vi "PTScanner.panel.vi"(0 "object ref":refnum<vi>, 5 "error in (no error)":errorcluster) -> ()   [LabVIEW 2014, in "PTScanner.lvlib"]
doc: "This is the front panel VI for the PTScanner class.\n\ndescriptionHelpStart\nThe PTScanner class has been designed to be used interactively by a normal user. The main aim of this class is to provide a possibility of multi-dimensional scan for any integer or floating-point single value among the CS system.\n\nAt first, user has to add values to be scanned and to organize them in the corresponding order. Each value is represented by several parameters:\n- object\n- \"set\" method (can have many parameters)\n- method parameters (with one of them to be scanned)\n- central point\n- \"minus\" and \"plus\" values (start point is a difference between \"central\" and \"minus\" values, stop point is a sum of \"central\" and \"plus\" respectively)\n- step size\n- call mode which means how will be realized the movement from one step to the next one. The check of nominal (from current step) and actual values conformity can be done in a simple mode (here you should know the corresponding service) or in a synchronous mode (assuming that the method has a feedback of excatly the same parameters as input parameters)\n- as an option one can input service address for the synchronization directly. Do it only if you know exactly what is it!!!\n\nAfter the list of values is formed you have to form the scan sequence. You can check the scan sequence by \"View -> Scan Table\" from the window menu (have to wait some time before the representation table will be formed). Now you can run your scan in two modes: single (sequence will be runned only once) and loop (sequence will be runned continuously).\n\nDelay is a delay time (in ms) between two steps.\ndescriptionHelpStop\n\nLicense Agreement for the PTScanner class:\n\nCopyright (C)\nMikhail Goncharov\nMax-Planck-Institut fuer Kernphysik\nSaupfercheckweg 1\n69117 Heidelberg\nGermany\n\nContact: mikhail.goncharov@mpi-hd.mpg.de\n\nThis program is free software; you can redistribute it and/or modify it under the terms of the GNU General Public License as published by the Free Software Foundation; either version 2 of the license, or (at your option) any later version.\n\nThis program is distributed in the hope that it will be useful, but WITHOUT ANY WARRANTY; without even the implied warranty of MERCHANTABILITY or FITNESS FOR A PARTICULAR PURPOSE. See the GNU General License for more details (http://www.gnu.org).\n\nLast update: 2-DEC-2010\n\n\nmenuHelpStart\nFile\n==\n- \"Load\" loads a list of values to be scanned. After that you have to form a scan.\n\n- \"Save/Save As\" saves the actual list of values.\n\n- \"Hide\" just hides this GUI (but it remains alive in the background).\n\n- \"Close\" closes this window and removes this process from the system.\n\nOperate\n=====\n- \"Start\" starts scan sequence. Awailable only after the sequence is formed.\n\n- \"Pause\" pauses current run. Awailable only during the running of the sequence.\n\n- \"Stop\" stops scan sequence.\n\n- \"Reset\" resets the scanner (sets the first step as a current and nulls all counters).\n\n- \"Reset Values\" sets all variables to their central values.\n\nView\n=====\n- \"Scan Table\" forms and shows the representation of the current formed scan sequence. If there are a lot of steps and values it could take some time so be patient =)\nmenuHelpStop"
uses:
  PTScanner.lvlib
  CSlibraries/UtilityLib/UtilityLib.helpType.ctl
  CSCore/CSSystem/CoreLib/CoreLib.string 2 byte array.vi
  CSCore/CSSystem/CSSystemLib/CSSystemLib.lvlib
  CSlibraries/UtilityLib/UtilityLib.lvlib
  _common/PTUtils/PTUtils.lvlib
  CSCore/CSSystem/CoreLib/CoreLib.lvlib
  CSCore/BaseProcess/BaseProcess.lvlib
  CSCore/BaseSM/BaseSM.lvlib
  CSCore/CSObj/CSObj.lvlib
panel:
  in  "Form step list":bool
  out "NewValue":i32
  out "state":string caption="State:"
  in  "Scan Delay":u32 caption="Delay:"
  out "Paused":bool
  in  "Set previous step":bool
  in  "Set next step":bool
  out "Current step":i32 caption="Step"
  in  "Mode":u16(ring) caption="Mode:" items=["Single", "Loop"]
  out "All done":bool caption="Done"
  out "Running":bool
  out "OldValue":i32
  in  "settings path":path caption="Settings file"
  out "Busy":bool
  out "ErrorString":string
  in  "tab":enum32{"Objects", "Scan Tree"}(tab)
  in  "object list":i32(listbox)
  out "Status Log":string
  out "Steps":string(tree)
  out "loop counter":i32
  out "error out":errorcluster
  # "ms"
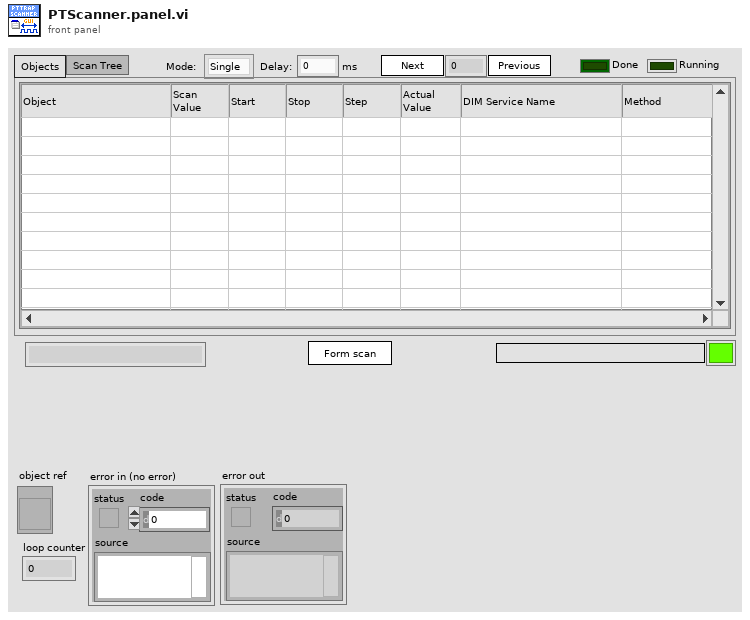
[diagram p1: front panel]
types:
  T1 = enum8{"Enabled", "Disabled", "Disabled and Grayed Out"}
  T2 = enum16{"open", "replace", "create", "open or create", "replace or create", "replace or create with confirmation"}
  T3 = typedef "UtilityLib.lvlib/UtilityLib.helpType.ctl" = enum16{"unknown", "menu", "description", "about", "special0", "special1", "special2"}
  T4 = typedef "BaseProcess.lvlib/BaseProcess.i attribute.ctl" = cluster{"EventStatus":string, "EventError":i32, "PresetEvtWatchD":i32, "PresetPdcWatchD":i32, "EventTimeout":i32, "PeriodicInterval":i32, "Interface":string[], "Address":string[], "Special":string[], "PeriodicError":i32, "PeriodicStatus":string, "SuperProc":string, "Descriptors":T5[], "CaseRef":refnum<vi>, "PdcRef":refnum<vi>, "Thread Ref":refnum<vi>, "eventErrorID":i32, "eventStatusID":i32, "periodicErrorID":i32, "periodicStatusID":i32, "pdcCtrID":i32}
  T5 = typedef "BaseProcess.lvlib/BaseProcess.descriptor definition.ctl" = cluster{"selector":string, "descriptor":T6}
  T6 = typedef "BaseProcess.lvlib/BaseProcess.descriptor string definition.ctl" = string
  T7 = typedef "PTScanner.lvlib/PTScanner.i attribute.ctl" = cluster{"Object cmds":T8[], "Steps":cluster{"Finished":bool, "cmd setup":T9[]}[], "curStep":i32, "DIM IDs":cluster{"AllFinished":i32, "Finished":i32, "curStep":i32, "nofSteps":i32, "NomValues":i32[], "1D-Min":i32, "1D-Max":i32, "Dimensions":i32, "MaxDimensions":i32, "ScanedDeviceNames":i32[]}, "All Finished":bool, "DIMs in use":string[], "Running":bool, "Scan Delay":u32, "loop":bool, "Paused":bool, "Formed":bool}
  T8 = typedef "PTScanner.lvlib/PTScanner.obj parameters.ctl" = cluster{"object":string, "DIM address":string, "method":string, "data descriptor":string, "method parameters":cluster{"Name":string, "Descr":string, "Value":string, "Value?":bool}[], "Call Mode":enum16{"Simple DIM", "Synchronous"}, "actValue":dbl, "Centroid":dbl, "Minus Delta":dbl, "Plus Delta":dbl, "increment":dbl, "DIM Status":cluster{"no link":bool, "quality":i32, "Time Stamp":timestamp}, "range":dbl, "DIMChannelIndex":i32}
  T9 = typedef "PTScanner.lvlib/PTScanner.step obj parameters.ctl" = cluster{"obj index":i32, "nomValue":dbl, "fulfilled":bool}
  T10 = cluster{"Name":string, "Descr":string, "Value":string, "Value?":bool}[]
  T11 = typedef "CoreDefs.rawDataType.ctl" = i8[]
  T12 = typedef "eventvkey.ctl" = enum16{"ASCII", "Enter", "Return", "Shift", "Ctrl", "Alt", "Cmd", "Opt", "Caps", "NumLock", "Clear", "Break", "Up", "Down", "Left", "Right", "Insert", "Delete", "Home", "End", "PageUp", "PageDown", "Escape", "Help", "Pause", "ScrollLock", "F1", "F2", "F3", "F4", "F5", "F6", "F7", "F8", "F9", "F10", "F11", "F12", "F13", "F14", "F15", "F16", "F17", "F18", "F19", "F20", "F21", "F22", "F23", "F24", "Play", "VolumeUp", "VolumeDown", "Mute", "Two Byte Char"}
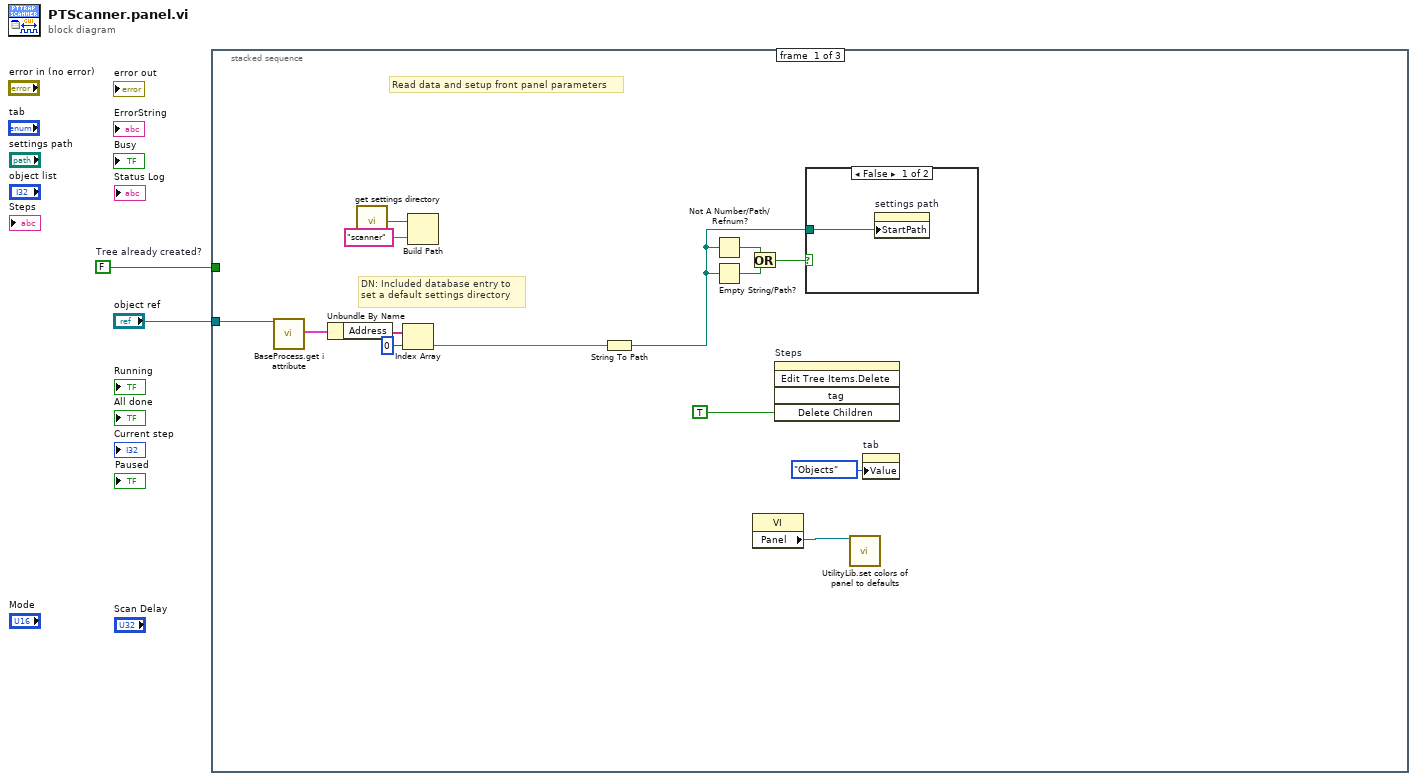
[diagram p0: block diagram]
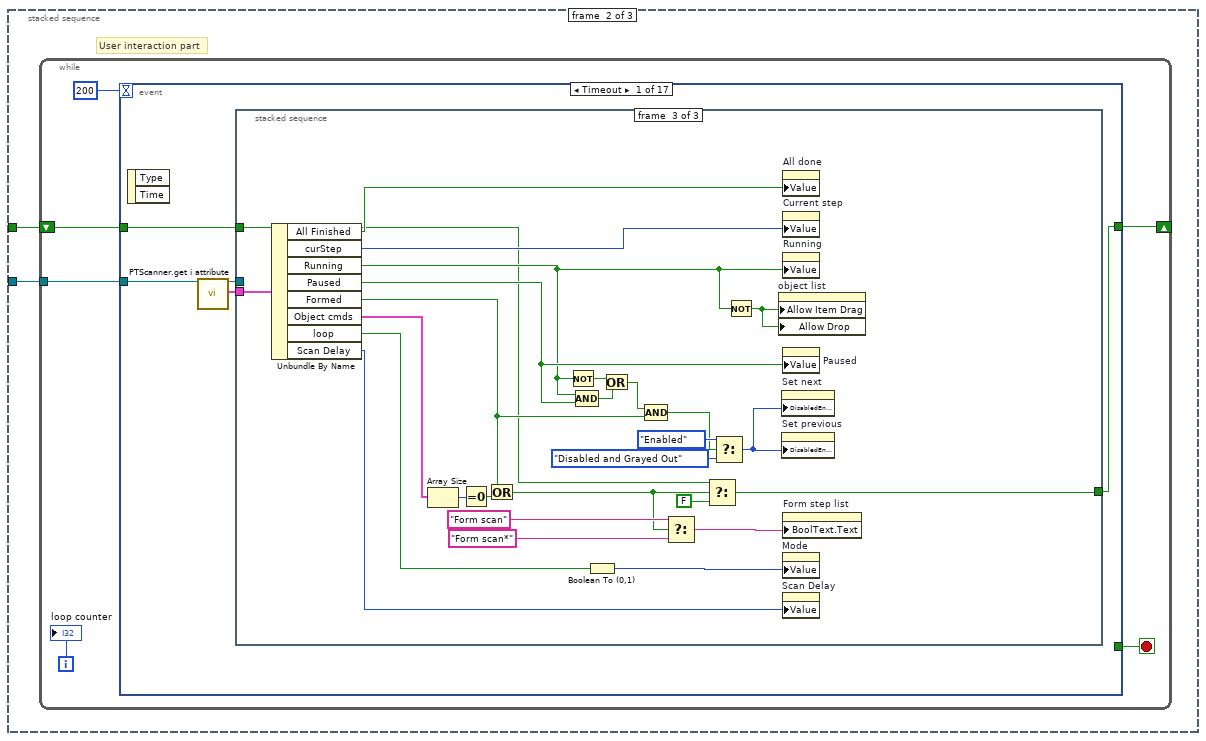
[diagram p3: hidden frame]
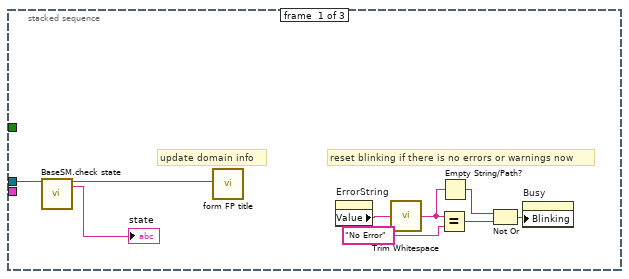
[diagram p4: hidden frame]
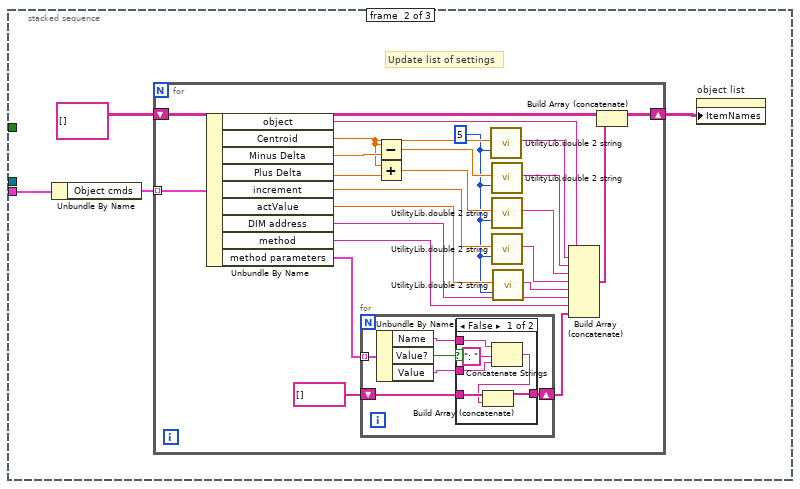
[diagram p5: hidden frame]
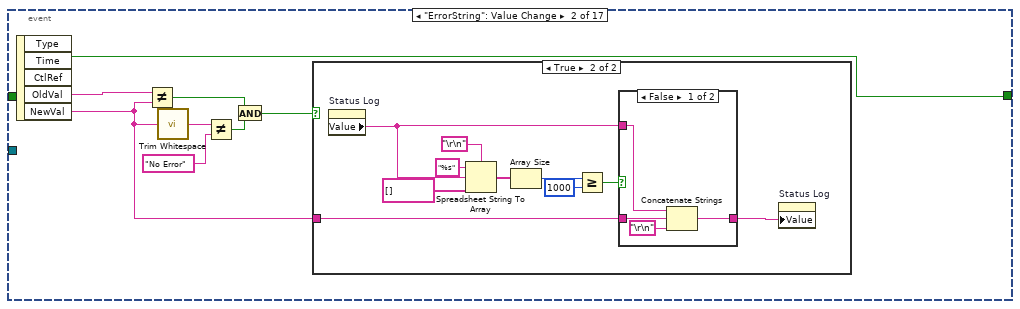
[diagram p7: hidden frame]
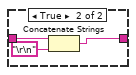
[diagram p9: hidden frame]
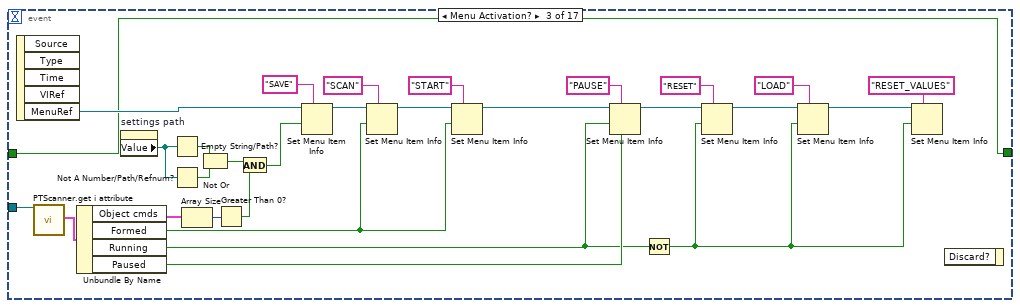
[diagram p10: hidden frame]
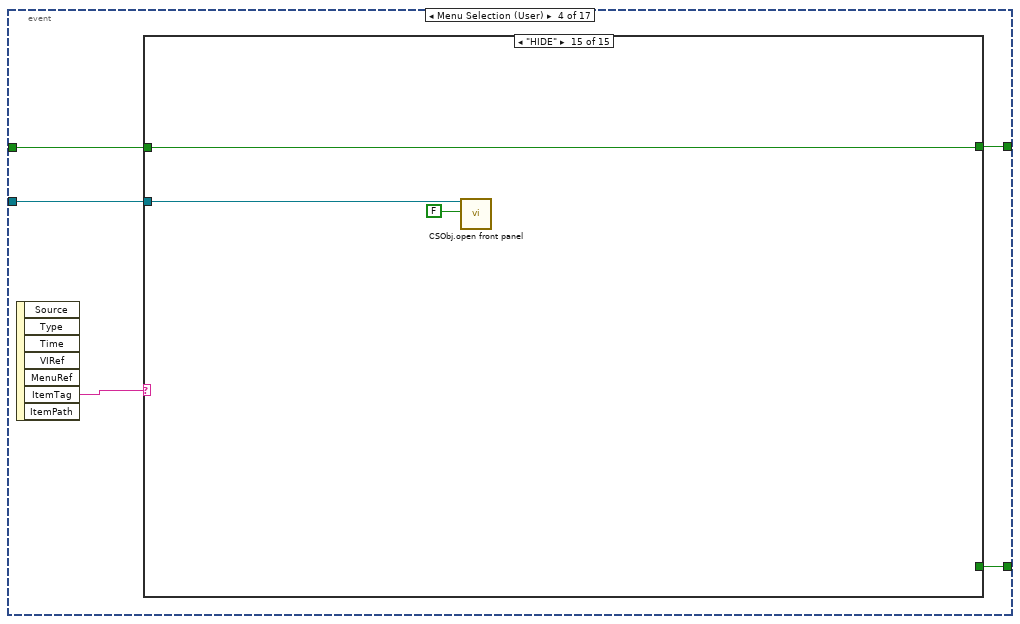
[diagram p11: hidden frame]
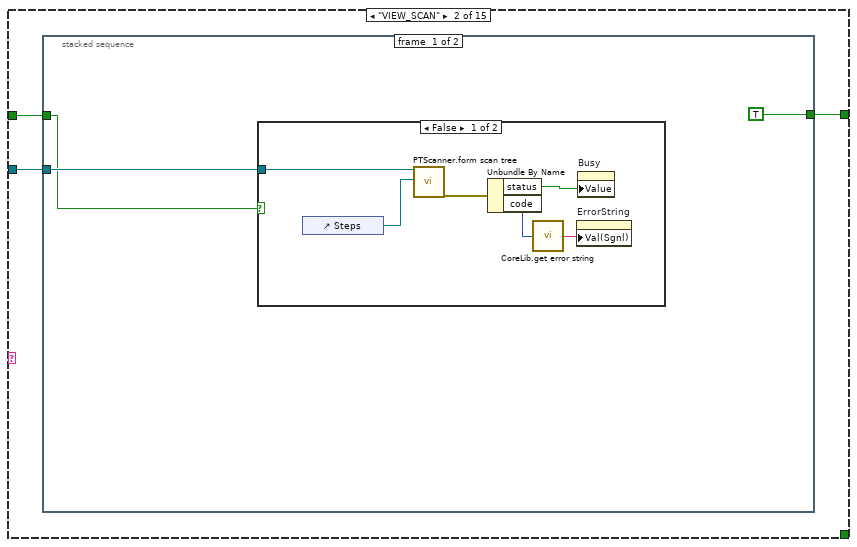
[diagram p13: hidden frame]
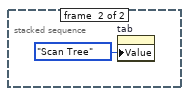
[diagram p15: hidden frame]
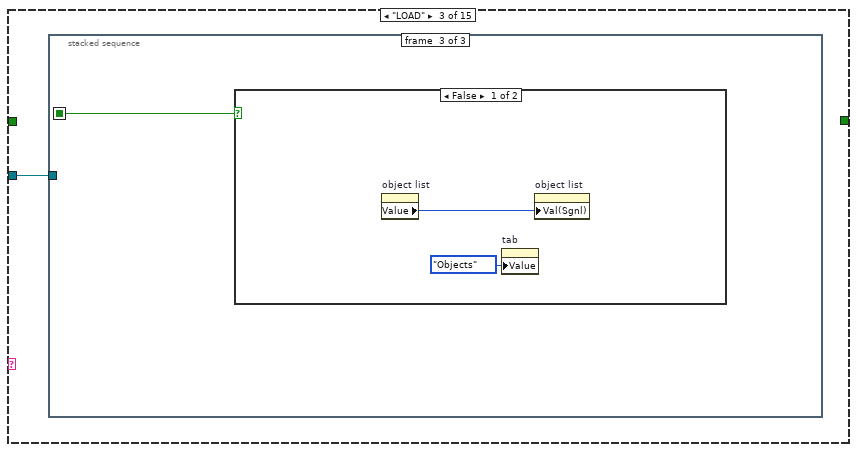
[diagram p16: hidden frame]
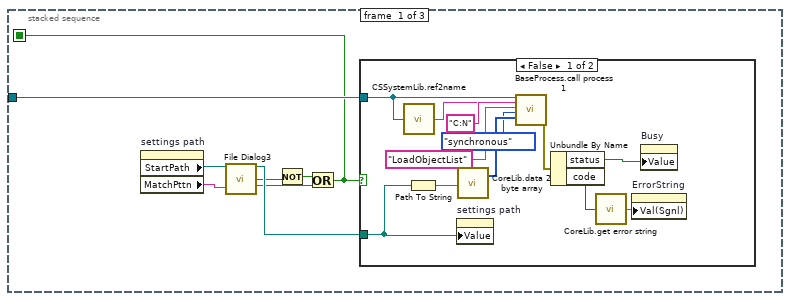
[diagram p17: hidden frame]
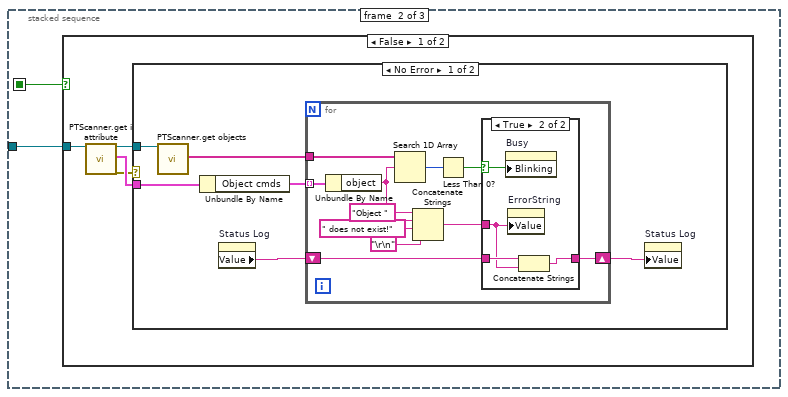
[diagram p19: hidden frame]
diagram:
  w1 = FALSE  # Tree already created?
  n1 = stacked-sequence {
    tunnel: "object ref" -> [w8 w19 w550]
    tunnel: w1 -> [_ w18 _]
    frame #0 {
      # "DN: Included database entry to\nset a default settings directory"
      # "Read data and setup front panel parameters"
      n2 = call "BaseProcess.get i attribute.vi"("i ref in"=w8) -> ("i attribute"=w7:T4)  [unwired: 16 in, 2 out]
      n3 = Unbundle By Name(w7) -> ("Address"=w6:string[])
      n4 = call "get settings directory.vi"() -> ("settings directory"=w12:path)
      n5 = Index Array(array=w6, index=0) -> (element=w4:string)
      n6 = Build Path(base path=w12, name or relative path="scanner") -> ()  [unwired: 1 out]
      n7 = String To Path(string=w4) -> (path=w3:path)
      n8 = Not A Number/Path/Refnum?(number/path/refnum=w3) -> (NaN/Path/Refnum?=w15:bool)
      n9 = Empty String/Path?(string/path=w3) -> (empty?=w14:bool)
      n10 = Or(x=w15, y=w14) -> (x .or. y?=w13:bool)
      n11 = property class="VI"() -> ("Panel"=w10:refnum<vi>)  [unwired: 2 in, 2 out]
      n12 = invoke on="Steps" class="Tree (strict)" method="Edit Tree Items.Delete"("Delete Children"=TRUE) -> ()  [unwired: 4 in, 5 out]
      n13 = case shown="False" w13 {
        tunnel: w3 -> [w17 _]
        frame False {
          n14 = property on="settings path" class="Path"("StartPath"=w17) -> ()  [unwired: 2 in, 2 out]
        }
        frame True {
        }
      }
      n15 = call "UtilityLib.set colors of panel to defaults.vi"("Front Panel"=w10) -> ()  [unwired: 18 in, 1 out]
      n16 = property on="tab" class="TabCtl (strict)"("Value"=enum32{"Objects", "Scan Tree"}."Objects" ("tab")) -> ()  [unwired: 2 in, 2 out]
    }
    frame #1 {
      # "User interaction part"
      n17 = while {
        tunnel: w19 -> [w25]
        shift-right: [w20] -> _
        shift-left: w18 -> [w21]
        i -> [w23]
        stop <- w22 stop-if-true
        n18 = event shown="[0] Timeout" {
          selector: _ -> [_ _ _ _ _ _ _ _ _ _ _ _ _ _ _ _ _]
          dyn-events: _ -> [_ _ _ _ _ _ _ _ _ _ _ _ _ _ _ _ _]
          timeout: 200 -> [_ _ _ _ _ _ _ _ _ _ _ _ _ _ _ _ _]
          tunnel: w25 -> [w30 _ w155 w164 w335 w353 _ w366 w398 w403 w468 w490 w517 w520 w528 w540 w547]
          tunnel: [_ _ _ w163 _ _ _ _ _ _ _ _ _ _ _ _ _] -> w22
          tunnel: w21 -> [w27 w107 w132 w162 w334 w342 w361 w364 w386 w402 w466 w489 _ w518 w526 w534 w546]
          tunnel: [w26 w107 w132 w161 TRUE w342 w361 w364 w386 w402 w466 w489 TRUE w518 w526 w534 w546] -> w20
          event Timeout {
            n19 = event-data() -> ()  [unwired: 1 in, 2 out]
            n20 = call "PTScanner.get i attribute.vi"("i ref in"=w30) -> ("i ref out"=w28:refnum<vi>, "i attribute"=w29:T7)  [unwired: 16 in, 1 out]
            n21 = stacked-sequence {
              tunnel: w29 -> [_ w41 w103]
              tunnel: w28 -> [w33 _ _]
              tunnel: w27 -> [_ _ w82]
              tunnel: [_ _ w80] -> w26
              frame #0 {
                # "update domain info"
                # "reset blinking if there is no errors or warnings now"
                n22 = call "BaseSM.check state.vi"("i ref in"=w33) -> ("i ref out"=w32:refnum<vi>, "actualState"=→"state":string)  [unwired: 13 in, 4 out]
                n23 = call "form FP title.vi"("object ref"=w32) -> ()  [unwired: 19 in]
                n24 = property on="ErrorString" class="Str"() -> ("Value"=w39:string)  [unwired: 2 in, 2 out]
                n25 = call <vilib>:"Trim Whitespace.vi"("string"=w39) -> ("trimmed string"=w37:string)  [unwired: 1 in]
                n26 = Equal?(x=w37, y="No Error") -> (x = y?=w35:bool)
                n27 = Empty String/Path?(string/path=w37) -> (empty?=w36:bool)
                n28 = Not Or(1:w35, 2:w36) -> (0:w34:bool)
                n29 = property on="Busy" class="Bool (strict)"("Blinking"=w34) -> ()  [unwired: 2 in, 2 out]
              }
              frame #1 {
                # "Update list of settings"
                n30 = Unbundle By Name(w41) -> ("Object cmds"=w42:T8[])
                n31 = for {
                  tunnel: w42 -> [w66] mode=indexing
                  shift-right: [w51] -> w40
                  shift-left: string[][] [] -> [w52]
                  w53 = u8 5
                  n32 = Unbundle By Name(w66) -> ("object"=w48:string, "Centroid"=w63:dbl, "Minus Delta"=w65:dbl, "Plus Delta"=w62:dbl, "increment"=w60:dbl, "actValue"=w59:dbl, "DIM address"=w54:string, "method"=w47:string, "method parameters"=w46:T10)
                  n33 = for {
                    tunnel: w46 -> [w72] mode=indexing
                    shift-right: [w70] -> w44
                    shift-left: string[] [] -> [w71]
                    n34 = Unbundle By Name(w72) -> ("Name"=w67:string, "Value?"=w68:bool, "Value"=w69:string)
                    n35 = case shown="False" w68 {
                      tunnel: w71 -> [w78 w79]
                      tunnel: [w77 w79] -> w70
                      tunnel: w67 -> [w76 _]
                      tunnel: w69 -> [w74 _]
                      frame False {
                        n36 = Concatenate Strings(w76, ": ", w74) -> (w73:string)
                        n37 = Build Array (concatenate)(w78, w73) -> (w77:string[])
                      }
                      frame True {
                      }
                    }
                  }
                  n38 = Subtract(x=w63, y=w65) -> (x-y=w64:dbl)
                  n39 = Add(x=w63, y=w62) -> (x+y=w61:dbl)
                  n40 = call "UtilityLib.double 2 string.vi"("Numeric"=w63, "length"=w53) -> ("String"=w49:string)  [unwired: 16 in, 1 out]
                  n41 = call "UtilityLib.double 2 string.vi"("Numeric"=w64, "length"=w53) -> ("String"=w58:string)  [unwired: 16 in, 1 out]
                  n42 = call "UtilityLib.double 2 string.vi"("Numeric"=w61, "length"=w53) -> ("String"=w57:string)  [unwired: 16 in, 1 out]
                  n43 = call "UtilityLib.double 2 string.vi"("Numeric"=w60, "length"=w53) -> ("String"=w56:string)  [unwired: 16 in, 1 out]
                  n44 = call "UtilityLib.double 2 string.vi"("Numeric"=w59, "length"=w53) -> ("String"=w55:string)  [unwired: 16 in, 1 out]
                  n45 = Build Array (concatenate)(w48, w49, w58, w57, w56, w55, w54, w47, w44) -> (w50:string[])
                  n46 = Build Array (concatenate)(w52, w50) -> (w51:string[][])
                }
                n47 = property on="object list" class="MCListbox (strict)"("ItemNames"=w40) -> ()  [unwired: 2 in, 2 out]
              }
              frame #2 {
                n48 = Unbundle By Name(w103) -> ("All Finished"=w92:bool, "curStep"=w93:i32, "Running"=w85:bool, "Paused"=w88:bool, "Formed"=w90:bool, "Object cmds"=w99:T8[], "loop"=w96:bool, "Scan Delay"=w94:u32)
                n49 = Array Size(array=w99) -> (size(s)=w98:i32)
                n50 = Equal To 0?(x=w98) -> (x = 0?=w97:bool)
                n51 = Or(x=w90, y=w97) -> (x .or. y?=w83:bool)
                n52 = Not(x=w85) -> (.not. x?=w89:bool)
                n53 = Compound Arithmetic op=AND(w85, w88) -> (w87:bool)
                n54 = Boolean To (0,1)(Boolean=w96) -> (0, 1=w95:i16)
                n55 = Or(x=w89, y=w87) -> (x .or. y?=w86:bool)
                n56 = Compound Arithmetic op=AND(w86, w90) -> (w91:bool)
                n57 = Select(t="Form scan", s=w83, f="Form scan*") -> (s? t:f=w102:string)
                n58 = Select(t=w82, s=w83, f=FALSE) -> (s? t:f=w80:bool)
                n59 = Select(t=T1."Enabled" ("Disabled"), s=w91, f=T1."Disabled and Grayed Out" ("Disabled")) -> (s? t:f=w106:T1)
                n60 = Not(x=w85) -> (.not. x?=w84:bool)
                n61 = property on="object list" class="MCListbox (strict)"("Allow Item Drag"=w84, "Allow Drop"=w84) -> ()  [unwired: 2 in, 2 out]
                n62 = property on="Set next" class="Bool"("DisabledEnum"=w106) -> ()  [unwired: 2 in, 2 out]
                n63 = property on="Set previous" class="Bool"("DisabledEnum"=w106) -> ()  [unwired: 2 in, 2 out]
                n64 = property on="All done" class="Bool (strict)"("Value"=w92) -> ()  [unwired: 2 in, 2 out]
                n65 = property on="Current step" class="DigNum (strict)"("Value"=w93) -> ()  [unwired: 2 in, 2 out]
                n66 = property on="Running" class="Bool (strict)"("Value"=w85) -> ()  [unwired: 2 in, 2 out]
                n67 = property on="Paused" class="Bool (strict)"("Value"=w88) -> ()  [unwired: 2 in, 2 out]
                n68 = property on="Form step list" class="Bool"("BoolText.Text"=w102) -> ()  [unwired: 2 in, 2 out]
                n69 = property on="Mode" class="Ring (strict)"("Value"=w95) -> ()  [unwired: 2 in, 2 out]
                n70 = property on="Scan Delay" class="DigNum (strict)"("Value"=w94) -> ()  [unwired: 2 in, 2 out]
              }
            }
          }
          event "ErrorString": Value Change {
            n71 = event-data() -> ("OldVal"=w114:string, "NewVal"=w111:string)  [unwired: 1 in, 3 out]
            n72 = Not Equal?(x=w114, y=w111) -> (x != y?=w109:bool)
            n73 = call <vilib>:"Trim Whitespace.vi"("string"=w111) -> ("trimmed string"=w113:string)  [unwired: 1 in]
            n74 = Not Equal?(x=w113, y="No Error") -> (x != y?=w110:bool)
            n75 = And(x=w109, y=w110) -> (x .and. y?=w108:bool)
            n76 = case shown="True" w108 {
              tunnel: w111 -> [_ w116]
              frame False {
              }
              frame True {
                n77 = property on="Status Log" class="Str"() -> ("Value"=w117:string)  [unwired: 2 in, 2 out]
                n78 = Spreadsheet String To Array(delimiter (Tab)="\r\n", format string="%s", spreadsheet string=w117, array type (2D Dbl)=string[] []) -> (array=w121:string[])
                n79 = Array Size(array=w121) -> (size(s)=w120:i32)
                n80 = Greater Or Equal?(x=w120, y=1000) -> (x >= y?=w118:bool)
                n81 = case shown="False" w118 {
                  tunnel: w117 -> [w128 _]
                  tunnel: w116 -> [w127 w130]
                  tunnel: [w125 w129] -> w115
                  frame False {
                    n82 = Concatenate Strings(w128, w127, "\r\n") -> (w125:string)
                  }
                  frame True {
                    n83 = Concatenate Strings(w130, "\r\n") -> (w129:string)
                  }
                }
                n84 = property on="Status Log" class="Str"("Value"=w115) -> ()  [unwired: 2 in, 2 out]
              }
            }
          }
          event Menu Activation? {
            n85 = event-data() -> ("MenuRef"=w160:refnum<k9>)  [unwired: 1 in, 4 out]
            n86 = call "PTScanner.get i attribute.vi"("i ref in"=w155) -> ("i attribute"=w154:T7)  [unwired: 16 in, 2 out]
            n87 = Unbundle By Name(w154) -> ("Object cmds"=w153:T8[], "Formed"=w134:bool, "Running"=w142:bool, "Paused"=w145:bool)
            n88 = property on="settings path" class="Path"() -> ("Value"=w156:path)  [unwired: 2 in, 2 out]
            n89 = Empty String/Path?(string/path=w156) -> (empty?=w158:bool)
            n90 = Not A Number/Path/Refnum?(number/path/refnum=w156) -> (NaN/Path/Refnum?=w157:bool)
            n91 = Array Size(array=w153) -> (size(s)=w152:i32)
            n92 = Not Or(1:w157, 2:w158) -> (0:w150:bool)
            n93 = Greater Than 0?(x=w152) -> (x > 0?=w151:bool)
            n94 = And(x=w150, y=w151) -> (x .and. y?=w149:bool)
            n95 = Set Menu Item Info(7:"SAVE", 9:w149, 11:w160) -> (3:w148:refnum<k9>)  [unwired: 4 in, 1 out]
            n96 = Set Menu Item Info(7:"SCAN", 9:w134, 11:w148) -> (3:w135:refnum<k9>)  [unwired: 4 in, 1 out]
            n97 = Set Menu Item Info(7:"START", 9:w134, 11:w135) -> (3:w133:refnum<k9>)  [unwired: 4 in, 1 out]
            n98 = Set Menu Item Info(6:w145, 7:"PAUSE", 9:w142, 11:w133) -> (3:w143:refnum<k9>)  [unwired: 3 in, 1 out]
            n99 = Not(x=w142) -> (.not. x?=w137:bool)
            n100 = Set Menu Item Info(7:"RESET", 9:w137, 11:w143) -> (3:w140:refnum<k9>)  [unwired: 4 in, 1 out]
            n101 = Set Menu Item Info(7:"LOAD", 9:w137, 11:w140) -> (3:w138:refnum<k9>)  [unwired: 4 in, 1 out]
            n102 = Set Menu Item Info(7:"RESET_VALUES", 9:w137, 11:w138) -> ()  [unwired: 4 in, 2 out]
            n103 = event-data() -> ()  [unwired: 2 in, 1 out]
          }
          event Menu Selection (User) {
            n104 = event-data() -> ("ItemTag"=w165:string)  [unwired: 1 in, 6 out]
            n105 = case shown="\"HIDE\"" w165 {
              tunnel: w164 -> [_ w169 w180 w237 w257 _ w282 w290 w302 w310 w318 _ _ _ w331]
              tunnel: [_ _ _ _ _ TRUE _ _ _ _ _ _ _ _ _] -> w163
              tunnel: w162 -> [w166 w168 _ w236 w255 w279 w281 w289 w297 w308 w316 w324 w326 w328 w330]
              tunnel: [w166 w167 _ w236 w255 w279 w281 w289 w297 w308 w316 w324 w326 w328 w330] -> w161
              frame "", Default {
              }
              frame "VIEW_SCAN" {
                n106 = stacked-sequence {
                  tunnel: w169 -> [w172 _]
                  tunnel: w168 -> [w171 _]
                  tunnel: [TRUE _] -> w167
                  frame #0 {
                    n107 = case shown="False" w171 {
                      tunnel: w172 -> [w177 _]
                      frame False {
                        n108 = control-ref of="Steps"() -> (w178:refnum<vi>)
                        n109 = call "PTScanner.form scan tree.vi"("VI Refnum"=w177, "Scan Tree Ref"=w178) -> ("error out"=w173:errorcluster)  [unwired: 16 in, 1 out]
                        n110 = Unbundle By Name(w173) -> ("status"=w176:bool, "code"=w174:i32)
                        n111 = call "CoreLib.get error string.vi"("Error Code"=w174) -> ("Error String"=w175:string)
                        n112 = property on="ErrorString" class="Str"("Val(Sgnl)"=w175) -> ()  [unwired: 2 in, 2 out]
                        n113 = property on="Busy" class="Bool (strict)"("Value"=w176) -> ()  [unwired: 2 in, 2 out]
                      }
                      frame True {
                      }
                    }
                  }
                  frame #1 {
                    n114 = property on="tab" class="TabCtl (strict)"("Value"=enum32{"Objects", "Scan Tree"}."Scan Tree" ("tab")) -> ()  [unwired: 2 in, 2 out]
                  }
                }
              }
              frame "LOAD" {
                n115 = stacked-sequence {
                  seq-local: [w182 _ _] -> [_ w201 w233]
                  tunnel: w180 -> [w186 w202 _]
                  frame #0 {
                    n116 = property on="settings path" class="Path"() -> ("StartPath"=w188:path, "MatchPttn"=w187:string)  [unwired: 2 in, 2 out]
                    n117 = call "File Dialog3"("start path"=w188, "pattern (all files)"=w187) -> ("selected path"=w185:path, "exists"=w181:bool, "cancelled"=w183:bool)  [unwired: 10 in, 1 out]
                    n118 = Not(x=w181) -> (.not. x?=w184:bool)
                    n119 = Or(x=w184, y=w183) -> (x .or. y?=w182:bool)
                    n120 = case shown="False" w182 {
                      tunnel: w186 -> [w192 _]
                      tunnel: w185 -> [w190 _]
                      frame False {
                        n121 = call "CSSystemLib.ref2name.vi"("obj refnum"=w192) -> ("name"=w193:string)
                        n122 = Path To String(path=w190) -> (string=w191:string)
                        n123 = property on="settings path" class="Path"("Value"=w190) -> ()  [unwired: 2 in, 2 out]
                        n124 = call-poly "CoreLib.data 2 byte array.vi"("string"=w191) -> ("byteArray out"=w194:T11)  [unwired: 18 in]
                        n125 = call "BaseProcess.call process 1.vi"("i ref in"=w192, "Object"=w193, "Selector"="LoadObjectList", "CallType"=enum16{"simple", "synchronous", "asynchronous"}."synchronous", "Data"=w194, "Data Descriptor"="C:N") -> ("error out"=w197:errorcluster)  [unwired: 11 in, 2 out]
                        n126 = Unbundle By Name(w197) -> ("status"=w200:bool, "code"=w198:i32)
                        n127 = call "CoreLib.get error string.vi"("Error Code"=w198) -> ("Error String"=w199:string)
                        n128 = property on="ErrorString" class="Str"("Val(Sgnl)"=w199) -> ()  [unwired: 2 in, 2 out]
                        n129 = property on="Busy" class="Bool (strict)"("Value"=w200) -> ()  [unwired: 2 in, 2 out]
                      }
                      frame True {
                      }
                    }
                  }
                  frame #1 {
                    n130 = case shown="False" w201 {
                      tunnel: w202 -> [w204 _]
                      frame False {
                        n131 = call "PTScanner.get i attribute.vi"("i ref in"=w204) -> ("i ref out"=w203:refnum<vi>, "i attribute"=w206:T7, "error out"=w205:errorcluster)  [unwired: 16 in]
                        n132 = case shown="No Error" w205 {
                          selector: w205 -> [_ w229]
                          tunnel: w206 -> [w210 _]
                          tunnel: w203 -> [w208 _]
                          frame No Error {
                            n133 = call "PTScanner.get objects.vi"("i ref in"=w208) -> ("objects"=w207:string[])  [unwired: 18 in]
                            n134 = Unbundle By Name(w210) -> ("Object cmds"=w209:T8[])
                            n135 = property on="Status Log" class="Str"() -> ("Value"=w212:string)  [unwired: 2 in, 2 out]
                            n136 = for {
                              tunnel: w209 -> [w222] mode=indexing
                              tunnel: w207 -> [w223]
                              shift-right: [w213] -> w211
                              shift-left: w212 -> [w215]
                              n137 = Unbundle By Name(w222) -> ("object"=w219:string)
                              n138 = Search 1D Array(1D array=w223, element=w219) -> (index of element=w221:i32)  [unwired: 1 in]
                              n139 = Concatenate Strings("Object ", w219, " does not exist!", "\r\n") -> (w214:string)
                              n140 = Less Than 0?(x=w221) -> (x < 0?=w220:bool)
                              n141 = case shown="True" w220 {
                                selector: w220 -> [_ w225]
                                tunnel: w215 -> [w224 w228]
                                tunnel: w214 -> [_ w227]
                                tunnel: [w224 w226] -> w213
                                frame False {
                                }
                                frame True {
                                n142 = property on="Busy" class="Bool (strict)"("Blinking"=w225) -> ()  [unwired: 2 in, 2 out]
                                n143 = property on="ErrorString" class="Str"("Value"=w227) -> ()  [unwired: 2 in, 2 out]
                                n144 = Concatenate Strings(w228, w227) -> (w226:string)
                                }
                              }
                            }
                            n145 = property on="Status Log" class="Str"("Value"=w211) -> ()  [unwired: 2 in, 2 out]
                          }
                          frame Error {
                            n146 = Unbundle By Name(w229) -> ("status"=w232:bool, "code"=w230:i32)
                            n147 = call "CoreLib.get error string.vi"("Error Code"=w230) -> ("Error String"=w231:string)
                            n148 = property on="ErrorString" class="Str"("Val(Sgnl)"=w231) -> ()  [unwired: 2 in, 2 out]
                            n149 = property on="Busy" class="Bool (strict)"("Value"=w232) -> ()  [unwired: 2 in, 2 out]
                          }
                        }
                      }
                      frame True {
                      }
                    }
                  }
                  frame #2 {
                    n150 = case shown="False" w233 {
                      frame False {
                        n151 = property on="object list" class="MCListbox (strict)"() -> ("Value"=w235:i32)  [unwired: 2 in, 2 out]
                        n152 = property on="tab" class="TabCtl (strict)"("Value"=enum32{"Objects", "Scan Tree"}."Objects" ("tab")) -> ()  [unwired: 2 in, 2 out]
                        n153 = property on="object list" class="MCListbox (strict)"("Val(Sgnl)"=w235) -> ()  [unwired: 2 in, 2 out]
                      }
                      frame True {
                      }
                    }
                  }
                }
              }
              frame "SAVE" {
                n154 = property on="settings path" class="Path"() -> ("Value"=w240:path)  [unwired: 2 in, 2 out]
                n155 = Open/Create/Replace File(file path (use dialog)=w240, operation (0:open)=T2."replace or create", access (0:read/write)=enum16{"read/write", "read-only", "write-only"}."read-only") -> (refnum out=w241:refnum<file>, cancelled=w243:bool)  [unwired: 3 in, 1 out]
                n156 = Close File(refnum=w241) -> (path=w242:path)  [unwired: 1 in, 1 out]
                n157 = case shown="False" w243 {
                  tunnel: w242 -> [w244 _]
                  tunnel: w237 -> [w246 _]
                  frame False {
                    n158 = call "CSSystemLib.ref2name.vi"("obj refnum"=w246) -> ("name"=w245:string)
                    n159 = Path To String(path=w244) -> (string=w247:string)
                    n160 = property on="settings path" class="Path"("Value"=w244) -> ()  [unwired: 2 in, 2 out]
                    n161 = call-poly "CoreLib.data 2 byte array.vi"("string"=w247) -> ("byteArray out"=w248:T11)  [unwired: 18 in]
                    n162 = call "BaseProcess.call process 2.vi"("i ref in"=w246, "Object"=w245, "Selector"="SaveObjectList", "Data Descriptor"="C:N", "Data"=w248) -> ("error out"=w251:errorcluster)  [unwired: 13 in, 1 out]
                    n163 = Unbundle By Name(w251) -> ("status"=w254:bool, "code"=w252:i32)
                    n164 = call "CoreLib.get error string.vi"("Error Code"=w252) -> ("Error String"=w253:string)
                    n165 = property on="Busy" class="Bool (strict)"("Value"=w254) -> ()  [unwired: 2 in, 2 out]
                    n166 = property on="ErrorString" class="Str"("Val(Sgnl)"=w253) -> ()  [unwired: 2 in, 2 out]
                  }
                  frame True {
                  }
                }
              }
              frame "SAVE_AS" {
                n167 = property on="settings path" class="Path"() -> ("StartPath"=w260:path, "MatchPttn"=w259:string)  [unwired: 2 in, 2 out]
                n168 = call "File Dialog4"("start path"=w260, "pattern (all files)"=w259) -> ("selected path"=w258:path, "cancelled"=w256:bool)  [unwired: 10 in, 2 out]
                n169 = case shown="False" w256 {
                  tunnel: w258 -> [w266 _]
                  tunnel: w257 -> [w267 _]
                  frame False {
                    n170 = Open/Create/Replace File(file path (use dialog)=w266, operation (0:open)=T2."replace or create with confirmation", access (0:read/write)=enum16{"read/write", "read-only", "write-only"}."read-only") -> (refnum out=w265:refnum<file>, cancelled=w263:bool)  [unwired: 3 in, 1 out]
                    n171 = Close File(refnum=w265) -> (path=w264:path)  [unwired: 1 in, 1 out]
                    n172 = case shown="False" w263 {
                      tunnel: w264 -> [w268 _]
                      tunnel: w267 -> [w270 _]
                      frame False {
                        n173 = call "CSSystemLib.ref2name.vi"("obj refnum"=w270) -> ("name"=w269:string)
                        n174 = Path To String(path=w268) -> (string=w271:string)
                        n175 = property on="settings path" class="Path"("Value"=w268) -> ()  [unwired: 2 in, 2 out]
                        n176 = call-poly "CoreLib.data 2 byte array.vi"("string"=w271) -> ("byteArray out"=w272:T11)  [unwired: 18 in]
                        n177 = call "BaseProcess.call process 2.vi"("i ref in"=w270, "Object"=w269, "Selector"="SaveObjectList", "Data Descriptor"="C:N", "Data"=w272) -> ("error out"=w275:errorcluster)  [unwired: 13 in, 1 out]
                        n178 = Unbundle By Name(w275) -> ("status"=w278:bool, "code"=w276:i32)
                        n179 = call "CoreLib.get error string.vi"("Error Code"=w276) -> ("Error String"=w277:string)
                        n180 = property on="ErrorString" class="Str"("Val(Sgnl)"=w277) -> ()  [unwired: 2 in, 2 out]
                        n181 = property on="Busy" class="Bool (strict)"("Value"=w278) -> ()  [unwired: 2 in, 2 out]
                      }
                      frame True {
                      }
                    }
                  }
                  frame True {
                  }
                }
              }
              frame "QUIT" {
              }
              frame "START" {
                n182 = call "CSSystemLib.ref2name.vi"("obj refnum"=w282) -> ("name"=w283:string)
                n183 = call "BaseProcess.call process 2.vi"("i ref in"=w282, "Object"=w283, "Selector"="Start") -> ("error out"=w284:errorcluster)  [unwired: 15 in, 1 out]
                n184 = Unbundle By Name(w284) -> ("status"=w287:bool, "code"=w285:i32)
                n185 = call "CoreLib.get error string.vi"("Error Code"=w285) -> ("Error String"=w286:string)
                n186 = property on="ErrorString" class="Str"("Val(Sgnl)"=w286) -> ()  [unwired: 2 in, 2 out]
                n187 = property on="Busy" class="Bool (strict)"("Value"=w287) -> ()  [unwired: 2 in, 2 out]
              }
              frame "STOP" {
                n188 = call "CSSystemLib.ref2name.vi"("obj refnum"=w290) -> ("name"=w291:string)
                n189 = call "BaseProcess.call process 2.vi"("i ref in"=w290, "Object"=w291, "Selector"="Stop") -> ("error out"=w292:errorcluster)  [unwired: 15 in, 1 out]
                n190 = Unbundle By Name(w292) -> ("status"=w295:bool, "code"=w293:i32)
                n191 = call "CoreLib.get error string.vi"("Error Code"=w293) -> ("Error String"=w294:string)
                n192 = property on="ErrorString" class="Str"("Val(Sgnl)"=w294) -> ()  [unwired: 2 in, 2 out]
                n193 = property on="Busy" class="Bool (strict)"("Value"=w295) -> ()  [unwired: 2 in, 2 out]
              }
              frame "PAUSE" {
                n194 = call "CSSystemLib.ref2name.vi"("obj refnum"=w302) -> ("name"=w303:string)
                n195 = property on="Paused" class="Bool (strict)"() -> ("Value"=w298:bool)  [unwired: 2 in, 2 out]
                n196 = Select(t="Start", s=w298, f="Pause") -> (s? t:f=w299:string)
                n197 = call "BaseProcess.call process 2.vi"("i ref in"=w302, "Object"=w303, "Selector"=w299) -> ("error out"=w304:errorcluster)  [unwired: 15 in, 1 out]
                n198 = Unbundle By Name(w304) -> ("status"=w307:bool, "code"=w305:i32)
                n199 = call "CoreLib.get error string.vi"("Error Code"=w305) -> ("Error String"=w306:string)
                n200 = property on="ErrorString" class="Str"("Val(Sgnl)"=w306) -> ()  [unwired: 2 in, 2 out]
                n201 = property on="Busy" class="Bool (strict)"("Value"=w307) -> ()  [unwired: 2 in, 2 out]
              }
              frame "RESET" {
                n202 = call "CSSystemLib.ref2name.vi"("obj refnum"=w310) -> ("name"=w311:string)
                n203 = call "BaseProcess.call process 2.vi"("i ref in"=w310, "Object"=w311, "Selector"="Reset") -> ("error out"=w312:errorcluster)  [unwired: 15 in, 1 out]
                n204 = Unbundle By Name(w312) -> ("status"=w315:bool, "code"=w313:i32)
                n205 = call "CoreLib.get error string.vi"("Error Code"=w313) -> ("Error String"=w314:string)
                n206 = property on="ErrorString" class="Str"("Val(Sgnl)"=w314) -> ()  [unwired: 2 in, 2 out]
                n207 = property on="Busy" class="Bool (strict)"("Value"=w315) -> ()  [unwired: 2 in, 2 out]
              }
              frame "RESET_VALUES" {
                n208 = call "CSSystemLib.ref2name.vi"("obj refnum"=w318) -> ("name"=w319:string)
                n209 = call "BaseProcess.call process 2.vi"("i ref in"=w318, "Object"=w319, "Selector"="SetCentralValues") -> ("error out"=w320:errorcluster)  [unwired: 15 in, 1 out]
                n210 = Unbundle By Name(w320) -> ("status"=w323:bool, "code"=w321:i32)
                n211 = call "CoreLib.get error string.vi"("Error Code"=w321) -> ("Error String"=w322:string)
                n212 = property on="ErrorString" class="Str"("Val(Sgnl)"=w322) -> ()  [unwired: 2 in, 2 out]
                n213 = property on="Busy" class="Bool (strict)"("Value"=w323) -> ()  [unwired: 2 in, 2 out]
              }
              frame "helpOnMenus" {
                n214 = call "UtilityLib.show help.vi"("helpType"=UtilityLib.helpType."menu") -> ()
              }
              frame "helpDescription" {
                n215 = call "UtilityLib.show help.vi"("helpType"=UtilityLib.helpType."description") -> ()
              }
              frame "helpAboutMe" {
                n216 = call "UtilityLib.show help.vi"("helpType"=UtilityLib.helpType."about") -> ()
              }
              frame "HIDE" {
                n217 = call "CSObj.open front panel.vi"("i ref in"=w331, "frontPanelOpen"=FALSE ("front panel open")) -> ()  [unwired: 16 in, 2 out]
              }
            }
          }
          event "tab": Value Change {
            n218 = event-data() -> ()  [unwired: 1 in, 6 out]
            n219 = case shown="False" w334 {
              tunnel: w335 -> [w339 _]
              frame False {
                n220 = control-ref of="Steps"() -> (w338:refnum<vi>)
                n221 = call "PTScanner.form scan tree.vi"("VI Refnum"=w339, "Scan Tree Ref"=w338) -> ("error out"=w341:errorcluster)  [unwired: 16 in, 1 out]
                n222 = Unbundle By Name(w341) -> ("status"=w337:bool, "code"=w340:i32)
                n223 = call "CoreLib.get error string.vi"("Error Code"=w340) -> ("Error String"=w336:string)
                n224 = property on="ErrorString" class="Str"("Val(Sgnl)"=w336) -> ()  [unwired: 2 in, 2 out]
                n225 = property on="Busy" class="Bool (strict)"("Value"=w337) -> ()  [unwired: 2 in, 2 out]
              }
              frame True {
              }
            }
          }
          event "Mode": Value Change {
            n226 = event-data() -> ("NewVal"=w354:u16)  [unwired: 1 in]
            n227 = Not Equal To 0?(x=w354) -> (x != 0?=w348:bool)
            n228 = call "PTScanner.get data to modify.vi"("i ref in"=w353, "ms timeout (10000)"=1000) -> ("i ref out"=w351:refnum<vi>, "i attribute"=w349:T7, "timed out"=w352:bool, "error out"=w350:errorcluster)  [unwired: 14 in]
            n229 = case shown="False" w352 {
              tunnel: w351 -> [w360 _]
              tunnel: w350 -> [w359 _]
              tunnel: w349 -> [w357 _]
              tunnel: w348 -> [w358 _]
              tunnel: [w355 _] -> w343
              frame False {
                n230 = Bundle By Name(cluster=w357, "loop"=w358) -> (w356:T7)
                n231 = call "PTScanner.set modified data.vi"("i ref in"=w360, "CLASS.i attribute"=w356, "error in (no error)"=w359) -> ("error out"=w355:errorcluster)  [unwired: 15 in, 1 out]
              }
              frame True {
              }
            }
            n232 = Unbundle By Name(w343) -> ("code"=w345:i32, "status"=w346:bool)
            n233 = local write "Busy"(w346) -> ()
            n234 = call "CoreLib.get error string.vi"("Error Code"=w345) -> ("Error String"=w344:string)
            n235 = property on="ErrorString" class="Str"("Val(Sgnl)"=w344) -> ()  [unwired: 2 in, 2 out]
          }
          event "object list": Value Change {
            n236 = event-data() -> ("OldVal"=→"OldValue":i32, "NewVal"=→"NewValue":i32)  [unwired: 1 in]
          }
          event "object list": Drag Ended {
            n237 = event-data() -> ()  [unwired: 1 in, 5 out]
            n238 = call "PTScanner.get data to modify.vi"("i ref in"=w366) -> ("i ref out"=w372:refnum<vi>, "i attribute"=w370:T7, "timed out"=w373:bool, "error out"=w371:errorcluster)  [unwired: 15 in]
            n239 = case shown="False" w373 {
              tunnel: w372 -> [w384 _]
              tunnel: w371 -> [w383 w385]
              tunnel: w370 -> [w382 _]
              tunnel: [w374 w385] -> w369
              frame False {
                n240 = Unbundle By Name(w382) -> ("Object cmds"=w380:T8[])
                n241 = local read "OldValue"() -> (w379:i32)
                n242 = local read "NewValue"() -> (w375:i32)
                n243 = Delete From Array(array=w380, index=w379) -> (deleted portion=w376:T8, array with subset deleted=w378:T8[])  [unwired: 1 in]
                n244 = Insert Into Array(array=w378, index=w375, new element=w376) -> (w377:T8[])
                n245 = Bundle By Name(cluster=w382, "Object cmds"=w377) -> (w381:T7)
                n246 = call "PTScanner.set modified data.vi"("i ref in"=w384, "CLASS.i attribute"=w381, "error in (no error)"=w383) -> ("error out"=w374:errorcluster)  [unwired: 15 in, 1 out]
              }
              frame True {
              }
            }
            n247 = Unbundle By Name(w369) -> ("code"=w367:i32, "status"=w368:bool)
            n248 = local write "Busy"(w368) -> ()
            n249 = call "CoreLib.get error string.vi"("Error Code"=w367) -> ("Error String"=w365:string)
            n250 = property on="ErrorString" class="Str"("Val(Sgnl)"=w365) -> ()  [unwired: 2 in, 2 out]
          }
          event "object list": Shortcut Menu Activation? {
            n251 = event-data() -> ("MenuRef"=w400:refnum<k9>)  [unwired: 1 in]
            n252 = call "PTScanner.get i attribute.vi"("i ref in"=w398) -> ("i attribute"=w397:T7)  [unwired: 16 in, 2 out]
            n253 = Unbundle By Name(w397) -> ("Running"=w390:bool)
            n254 = Not(x=w390) -> (.not. x?=w388:bool)
            n255 = property on="object list" class="MCListbox (strict)"() -> ("Value"=w399:i32)  [unwired: 2 in, 2 out]
            n256 = Greater Or Equal To 0?(x=w399) -> (x >= 0?=w389:bool)
            n257 = And(x=w389, y=w388) -> (x .and. y?=w387:bool)
            n258 = Set Menu Item Info(7:"EDIT", 9:w387, 11:w400) -> (3:w393:refnum<k9>)  [unwired: 4 in, 1 out]
            n259 = Set Menu Item Info(7:"ADD", 9:w388, 11:w393) -> (3:w392:refnum<k9>)  [unwired: 4 in, 1 out]
            n260 = Set Menu Item Info(7:"DELETE", 9:w388, 11:w392) -> (3:w391:refnum<k9>)  [unwired: 4 in, 1 out]
            n261 = Set Menu Item Info(7:"CLEAR_LIST", 9:w388, 11:w391) -> ()  [unwired: 4 in, 2 out]
            n262 = event-data() -> ()  [unwired: 2 in, 1 out]
          }
          event "object list": Shortcut Menu Selection (User) {
            n263 = event-data() -> ("ItemTag"=w404:string)  [unwired: 1 in]
            n264 = case shown="\"CLEAR_LIST\"" w404 {
              tunnel: w403 -> [w408 w416 w438 w454]
              frame "ADD" {
                n265 = call "PTScanner.dialog edit object.vi"("object ref"=w408, "new"=TRUE) -> ("object ref out"=w405:refnum<vi>, "Parameters Out"=w407:T8, "changed"=w406:bool)  [unwired: 15 in]
                n266 = case shown="True" w406 {
                  tunnel: w405 -> [_ w411]
                  tunnel: w407 -> [_ w410]
                  frame False {
                  }
                  frame True {
                    n267 = call "PTScanner.add object.vi"("i ref in"=w411, "Parameters"=w410) -> ("error out"=w414:errorcluster)  [unwired: 16 in, 1 out]
                    n268 = Unbundle By Name(w414) -> ("code"=w415:i32, "status"=w413:bool)
                    n269 = local write "Busy"(w413) -> ()
                    n270 = call "CoreLib.get error string.vi"("Error Code"=w415) -> ("Error String"=w412:string)
                    n271 = property on="ErrorString" class="Str"("Val(Sgnl)"=w412) -> ()  [unwired: 2 in, 2 out]
                  }
                }
              }
              frame "EDIT", Default {
                n272 = call "PTScanner.get i attribute.vi"("i ref in"=w416) -> ("i ref out"=w423:refnum<vi>, "i attribute"=w422:T7)  [unwired: 16 in, 1 out]
                n273 = Unbundle By Name(w422) -> ("Object cmds"=w419:T8[])
                n274 = property on="object list" class="MCListbox (strict)"() -> ("Value"=w421:i32)  [unwired: 2 in, 2 out]
                n275 = Array Size(array=w419) -> (size(s)=w418:i32)
                n276 = In Range and Coerce(upper limit=w418, x=w421, lower limit=0) -> (coerced(x)=w417:i32)  [unwired: 1 out]
                n277 = case shown="1, Default" w418 {
                  tunnel: w423 -> [_ w424]
                  tunnel: w419 -> [_ w429]
                  tunnel: w417 -> [_ w428]
                  frame 0 {
                  }
                  frame 1, Default {
                    n278 = Index Array(array=w429, index=w428) -> (element=w426:T8)
                    n279 = call "PTScanner.dialog edit object.vi"("object ref"=w424, "Parameters In"=w426, "new"=FALSE) -> ("Parameters Out"=w425:T8, "changed"=w427:bool)  [unwired: 14 in, 1 out]
                    n280 = case shown="True" w427 {
                      tunnel: w425 -> [_ w433]
                      tunnel: w424 -> [_ w432]
                      tunnel: w428 -> [_ w431]
                      frame False {
                      }
                      frame True {
                        n281 = call "PTScanner.edit object.vi"("i ref in"=w432, "Parameters"=w433, "index"=w431) -> ("error out"=w436:errorcluster)  [unwired: 15 in, 1 out]
                        n282 = Unbundle By Name(w436) -> ("code"=w437:i32, "status"=w435:bool)
                        n283 = local write "Busy"(w435) -> ()
                        n284 = call "CoreLib.get error string.vi"("Error Code"=w437) -> ("Error String"=w434:string)
                        n285 = property on="ErrorString" class="Str"("Val(Sgnl)"=w434) -> ()  [unwired: 2 in, 2 out]
                      }
                    }
                  }
                }
              }
              frame "DELETE" {
                n286 = stacked-sequence {
                  tunnel: w438 -> [w440 w445]
                  frame #0 {
                    n287 = property on="object list" class="MCListbox (strict)"() -> ("Value"=w441:i32)  [unwired: 2 in, 2 out]
                    n288 = call "PTScanner.remove object.vi"("i ref in"=w440, "index"=w441) -> ("error out"=w444:errorcluster)  [unwired: 16 in, 1 out]
                    n289 = Unbundle By Name(w444) -> ("code"=w443:i32, "status"=w442:bool)
                    n290 = local write "Busy"(w442) -> ()
                    n291 = call "CoreLib.get error string.vi"("Error Code"=w443) -> ("Error String"=w439:string)
                    n292 = property on="ErrorString" class="Str"("Val(Sgnl)"=w439) -> ()  [unwired: 2 in, 2 out]
                  }
                  frame #1 {
                    n293 = call "PTScanner.get i attribute.vi"("i ref in"=w445) -> ("i attribute"=w446:T7)  [unwired: 16 in, 2 out]
                    n294 = Unbundle By Name(w446) -> ("Object cmds"=w452:T8[])
                    n295 = Array Size(array=w452) -> (size(s)=w451:i32)
                    n296 = property on="object list" class="MCListbox (strict)"() -> ("Value"=w447:i32)  [unwired: 2 in, 2 out]
                    n297 = Decrement(x=w451) -> (x-1=w450:i32)
                    n298 = In Range and Coerce(upper limit=w450, x=w447, lower limit=0) -> (In Range?=w448:bool)  [unwired: 1 out]
                    n299 = case shown="True" w448 {
                      tunnel: w447 -> [_ w453]
                      frame False {
                      }
                      frame True {
                        n300 = property on="object list" class="MCListbox (strict)"("Val(Sgnl)"=w453) -> ()  [unwired: 2 in, 2 out]
                      }
                    }
                  }
                }
              }
              frame "CLEAR_LIST" {
                n301 = Two Button Dialog(message="Clear object list?", 1:"No", 2:"Yes") -> (T button?=w455:bool)
                n302 = case shown="True" w455 {
                  tunnel: w454 -> [_ w459]
                  frame False {
                  }
                  frame True {
                    n303 = call "CSSystemLib.ref2name.vi"("obj refnum"=w459) -> ("name"=w460:string)
                    n304 = call "BaseProcess.call process 2.vi"("i ref in"=w459, "Object"=w460, "Selector"="ClearObjectList") -> ("error out"=w461:errorcluster)  [unwired: 15 in, 1 out]
                    n305 = Unbundle By Name(w461) -> ("status"=w464:bool, "code"=w462:i32)
                    n306 = call "CoreLib.get error string.vi"("Error Code"=w462) -> ("Error String"=w463:string)
                    n307 = property on="ErrorString" class="Str"("Val(Sgnl)"=w463) -> ()  [unwired: 2 in, 2 out]
                    n308 = property on="Busy" class="Bool (strict)"("Value"=w464) -> ()  [unwired: 2 in, 2 out]
                  }
                }
              }
            }
          }
          event "object list": Double Click {
            n309 = event-data() -> ()  [unwired: 1 in, 3 out]
            n310 = property on="object list" class="MCListbox (strict)"() -> ("Value"=w467:i32)  [unwired: 2 in, 2 out]
            n311 = case shown="0, Default" w467 {
              selector: w467 -> [w469 _]
              tunnel: w468 -> [w470 _]
              frame 0, Default {
                n312 = call "PTScanner.get i attribute.vi"("i ref in"=w470) -> ("i ref out"=w474:refnum<vi>, "i attribute"=w473:T7)  [unwired: 16 in, 1 out]
                n313 = Unbundle By Name(w473) -> ("Object cmds"=w472:T8[])
                n314 = Array Size(array=w472) -> (size(s)=w471:i32)
                n315 = case shown="1, Default" w471 {
                  tunnel: w474 -> [_ w475]
                  tunnel: w472 -> [_ w480]
                  tunnel: w469 -> [_ w479]
                  frame 0 {
                  }
                  frame 1, Default {
                    n316 = Index Array(array=w480, index=w479) -> (element=w477:T8)
                    n317 = call "PTScanner.dialog edit object.vi"("object ref"=w475, "Parameters In"=w477, "new"=FALSE) -> ("Parameters Out"=w476:T8, "changed"=w478:bool)  [unwired: 14 in, 1 out]
                    n318 = case shown="True" w478 {
                      tunnel: w476 -> [_ w484]
                      tunnel: w475 -> [_ w483]
                      tunnel: w479 -> [_ w482]
                      frame False {
                      }
                      frame True {
                        n319 = call "PTScanner.edit object.vi"("i ref in"=w483, "Parameters"=w484, "index"=w482) -> ("error out"=w487:errorcluster)  [unwired: 15 in, 1 out]
                        n320 = Unbundle By Name(w487) -> ("code"=w488:i32, "status"=w486:bool)
                        n321 = local write "Busy"(w486) -> ()
                        n322 = call "CoreLib.get error string.vi"("Error Code"=w488) -> ("Error String"=w485:string)
                        n323 = property on="ErrorString" class="Str"("Val(Sgnl)"=w485) -> ()  [unwired: 2 in, 2 out]
                      }
                    }
                  }
                }
              }
              frame -1 {
              }
            }
          }
          event "object list": Key Down? {
            n324 = event-data() -> ("VKey"=w492:T12)  [unwired: 1 in]
            n325 = case shown="\"Delete\"" w492 {
              tunnel: [TRUE _] -> w491
              tunnel: w490 -> [_ w494]
              frame "ASCII", Default {
              }
              frame "Delete" {
                n326 = stacked-sequence {
                  tunnel: w494 -> [w496 w501]
                  frame #0 {
                    n327 = property on="object list" class="MCListbox (strict)"() -> ("Value"=w497:i32)  [unwired: 2 in, 2 out]
                    n328 = call "PTScanner.remove object.vi"("i ref in"=w496, "index"=w497) -> ("error out"=w500:errorcluster)  [unwired: 16 in, 1 out]
                    n329 = Unbundle By Name(w500) -> ("code"=w499:i32, "status"=w498:bool)
                    n330 = local write "Busy"(w498) -> ()
                    n331 = call "CoreLib.get error string.vi"("Error Code"=w499) -> ("Error String"=w495:string)
                    n332 = property on="ErrorString" class="Str"("Val(Sgnl)"=w495) -> ()  [unwired: 2 in, 2 out]
                  }
                  frame #1 {
                    n333 = call "PTScanner.get i attribute.vi"("i ref in"=w501) -> ("i attribute"=w502:T7)  [unwired: 16 in, 2 out]
                    n334 = Unbundle By Name(w502) -> ("Object cmds"=w508:T8[])
                    n335 = Array Size(array=w508) -> (size(s)=w507:i32)
                    n336 = property on="object list" class="MCListbox (strict)"() -> ("Value"=w503:i32)  [unwired: 2 in, 2 out]
                    n337 = Decrement(x=w507) -> (x-1=w506:i32)
                    n338 = In Range and Coerce(upper limit=w506, x=w503, lower limit=0) -> (In Range?=w504:bool)  [unwired: 1 out]
                    n339 = case shown="True" w504 {
                      tunnel: w503 -> [_ w509]
                      frame False {
                      }
                      frame True {
                        n340 = property on="object list" class="MCListbox (strict)"("Val(Sgnl)"=w509) -> ()  [unwired: 2 in, 2 out]
                      }
                    }
                  }
                }
              }
            }
            n341 = event-data("Discard?"=w491) -> ()  [unwired: 6 in, 1 out]
          }
          event "Form step list": Value Change {
            n342 = event-data() -> ()  [unwired: 1 in, 6 out]
            n343 = call "CSSystemLib.ref2name.vi"("obj refnum"=w517) -> ("name"=w511:string)
            n344 = call "BaseProcess.call process 2.vi"("i ref in"=w517, "Object"=w511, "Selector"="FormScan") -> ("error out"=w512:errorcluster)  [unwired: 15 in, 1 out]
            n345 = Unbundle By Name(w512) -> ("status"=w515:bool, "code"=w513:i32)
            n346 = call "CoreLib.get error string.vi"("Error Code"=w513) -> ("Error String"=w514:string)
            n347 = property on="ErrorString" class="Str"("Val(Sgnl)"=w514) -> ()  [unwired: 2 in, 2 out]
            n348 = property on="Busy" class="Bool (strict)"("Value"=w515) -> ()  [unwired: 2 in, 2 out]
          }
          event "Set next step": Value Change {
            n349 = event-data() -> ()  [unwired: 1 in, 6 out]
            n350 = call "CSSystemLib.ref2name.vi"("obj refnum"=w520) -> ("name"=w519:string)
            n351 = call "BaseProcess.call process 2.vi"("i ref in"=w520, "Object"=w519, "Selector"="SetNextStep") -> ("error out"=w521:errorcluster)  [unwired: 15 in, 1 out]
            n352 = Unbundle By Name(w521) -> ("status"=w524:bool, "code"=w522:i32)
            n353 = call "CoreLib.get error string.vi"("Error Code"=w522) -> ("Error String"=w523:string)
            n354 = property on="ErrorString" class="Str"("Val(Sgnl)"=w523) -> ()  [unwired: 2 in, 2 out]
            n355 = property on="Busy" class="Bool (strict)"("Value"=w524) -> ()  [unwired: 2 in, 2 out]
          }
          event "Set previous step": Value Change {
            n356 = event-data() -> ()  [unwired: 1 in, 6 out]
            n357 = call "CSSystemLib.ref2name.vi"("obj refnum"=w528) -> ("name"=w527:string)
            n358 = call "BaseProcess.call process 2.vi"("i ref in"=w528, "Object"=w527, "Selector"="SetPreviousStep") -> ("error out"=w529:errorcluster)  [unwired: 15 in, 1 out]
            n359 = Unbundle By Name(w529) -> ("status"=w532:bool, "code"=w530:i32)
            n360 = call "CoreLib.get error string.vi"("Error Code"=w530) -> ("Error String"=w531:string)
            n361 = property on="ErrorString" class="Str"("Val(Sgnl)"=w531) -> ()  [unwired: 2 in, 2 out]
            n362 = property on="Busy" class="Bool (strict)"("Value"=w532) -> ()  [unwired: 2 in, 2 out]
          }
          event "Scan Delay": Value Change {
            n363 = event-data() -> ("NewVal"=w535:u32)  [unwired: 1 in]
            n364 = call "PTScanner.get data to modify.vi"("i ref in"=w540) -> ("i ref out"=w537:refnum<vi>, "i attribute"=w539:T7, "timed out"=w538:bool, "error out"=w536:errorcluster)  [unwired: 15 in]
            n365 = case shown="False" w538 {
              tunnel: w539 -> [w545 _]
              tunnel: w537 -> [w543 _]
              tunnel: w536 -> [w542 _]
              tunnel: w535 -> [w541 _]
              frame False {
                n366 = Bundle By Name(cluster=w545, "Scan Delay"=w541) -> (w544:T7)
                n367 = call "PTScanner.set modified data.vi"("i ref in"=w543, "CLASS.i attribute"=w544, "error in (no error)"=w542) -> ()  [unwired: 15 in, 2 out]
              }
              frame True {
              }
            }
          }
          event Panel Close? {
            n368 = event-data() -> ()  [unwired: 1 in, 4 out]
            n369 = call "CSObj.open front panel.vi"("i ref in"=w547, "frontPanelOpen"=FALSE ("front panel open")) -> ()  [unwired: 16 in, 2 out]
            n370 = event-data() -> ()  [unwired: 2 in, 1 out]
          }
        }
        "loop counter" <- w23
      }
    }
    frame #2 {
      # "Close panel - run GOG destructor"
      n371 = call "destroy this.vi"("i ref in"=w550, "close FP first"=TRUE) -> ()  [unwired: 17 in, 1 out]
    }
  }
